vi "Load Plugins.vi"(8 "error in (no error)":errorcluster, 11 "TargetPluginManager in":refnum<class "PlatformPluginManager.lvclass">) -> (0 "error out":errorcluster, 3 "TargetPluginManager out":refnum<class "PlatformPluginManager.lvclass">)   [LabVIEW 2020, in "PicoG-Core.lvlib" / "PlatformPluginManager.lvclass"]
uses:
  PlatformPluginManager.lvclass
  PlatformPluginManager.lvclass/PlatformPluginManager.ctl
  DeployPlatform/DeployPlatform.lvclass
  <vilib>/Utility/LVLibp/NI_PackedLibraryUtility.lvlib
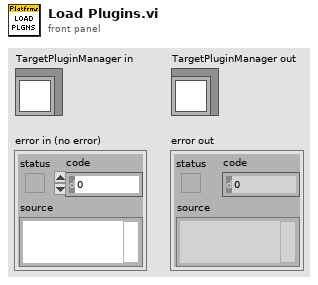
[diagram p1: front panel]
types:
  T1 = typedef "PicoG-Core.lvlib/PlatformPluginManager.lvclass/Ref Data.ctl" = cluster{"Platforms":refnum<class "DeployPlatform.lvclass">[], "Last Platform":refnum<class "DeployPlatform.lvclass">, "Last Resource":refnum<class "DeployResource.lvclass">}
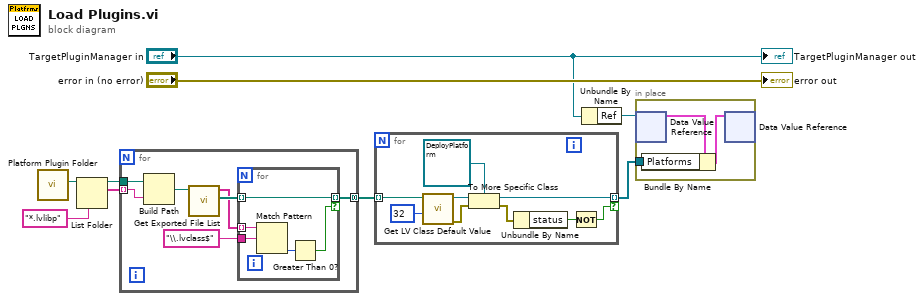
[diagram p0: block diagram]
diagram:
  n1 = call "Platform Plugin Folder.vi"() -> ("Path"=w4:path)  [unwired: 11 in]
  n2 = List Folder(path=w4, pattern="*.lvlibp") -> (path out=w7:path, filenames=w6:string[])  [unwired: 2 in, 2 out]
  n3 = for {
    tunnel: w7 -> [w16]
    tunnel: w6 -> [w15] mode=indexing
    tunnel: [w10] -> w5 mode=concatenating
    n4 = Build Path(base path=w16, name or relative path=w15) -> (appended path=w14:path)
    n5 = call <vilib>:"Get Exported File List.vi"("packed library path"=w14) -> ("paths"=w13:path[], "qualified names"=w12:string[])  [unwired: 8 in, 1 out]
    n6 = for {
      tunnel: w13 -> [w19] mode=indexing
      tunnel: w12 -> [w21] mode=indexing
      tunnel: "\\.lvclass$" ("regular expression") -> [w20]
      tunnel: [w19] -> w10 mode=indexing if=w17
      n7 = Match Pattern(string=w21, regular expression=w20) -> (offset past match=w18:i32)  [unwired: 1 in, 3 out]
      n8 = Greater Than 0?(x=w18) -> (x > 0?=w17:bool)
    }
  }
  n9 = for {
    tunnel: w5 -> [w30] mode=indexing
    tunnel: [w26] -> w1 mode=indexing if=w23
    n10 = call <vilib>:"Get LV Class Default Value.vi"("options"=u32 32, "class path"=w30) -> ("error out"=w28:errorcluster, "object"=w29:refnum<class>)  [unwired: 8 in]
    n11 = To More Specific Class(target class=refnum<class "DeployPlatform.lvclass"> refnum ("PicoG-Core:DeployTarget"), reference=w29, error in=w28) -> (specific class reference=w26:refnum<class "DeployPlatform.lvclass">, error out=w25:errorcluster)
    n12 = Unbundle By Name(w25) -> ("status"=w24:bool)
    n13 = Not(x=w24) -> (.not. x?=w23:bool)
  }
  n14 = Unbundle By Name("TargetPluginManager in") -> ("Ref"=w3:refnum<data-value>)
  n15 = in-place {
    in-place-border: w1 -> [w31]
    n16 = in-place-dvr #1(w3) -> (w33:T1)  [unwired: 1 out]
    n17 = Bundle By Name(cluster=w33, "Platforms"=w31) -> (w32:T1)
    n18 = in-place-dvr #1(w32) -> ()  [unwired: 2 out]
  }
  "error out" <- "error in (no error)"
  "TargetPluginManager out" <- "TargetPluginManager in"
